vi "ReadTorque-sub.vi"(0 "Torque Setpoint":dbl=1.0 format="%#_13g", 1 "Test Time":dbl, 9 "index 2":i32, 12 "State 2":bool, 13 "State 3":bool) -> (3 "Encoder":dbl[](array[numeric]), 4 "Torque":dbl[](array[numeric]), 5 "Torque":cluster{dbl, dbl}[](array[cluster]), 6 "RPMValue":i32, 8 "Torque vs. Angle":cluster{dbl, dbl}[](array[cluster]), 10 "rpm":cluster{dbl, dbl}[](array[cluster]), 11 "Voltage":cluster{dbl, "voltage out":dbl}[](array[cluster]), 15 "error out":errorcluster)   [LabVIEW 2015]
uses:
  <vilib>/Platform/TimedLoop/XDataNode/timing_clust.ctl
  <vilib>/Platform/TimedLoop/XDataNode/nitl_modes.ctl
  <vilib>/Platform/TimedLoop/XDataNode/wakeup.ctl
  C:/Program Files (x86)/National Instruments/LabVIEW 2015/FUTEK USB DLL.dll
  FUTEK USB DLL.dll
  <vilib>/platform/TimedLoop/XDataNode/XDataNode.xnode
  <vilib>/Platform/TimedLoop/XDataNode/XDNodeRunTimeDep.lvlib
panel:
  out "Array":cluster{dbl, "Torque Error":dbl}[](array[cluster])
  in  "FirstFound":bool=TRUE
  in  "Address":string="1"
  out "Get ADC Sampling RAte 2":string
  out "Get_Decimal Point":string
  out "Get_Fullscale_Load":string
  out "Get_Fullscale_Value":string
  out "Get_Offset_Load":string
  out "Get_Offset_Value":string
  out "get Rotation values 2":string
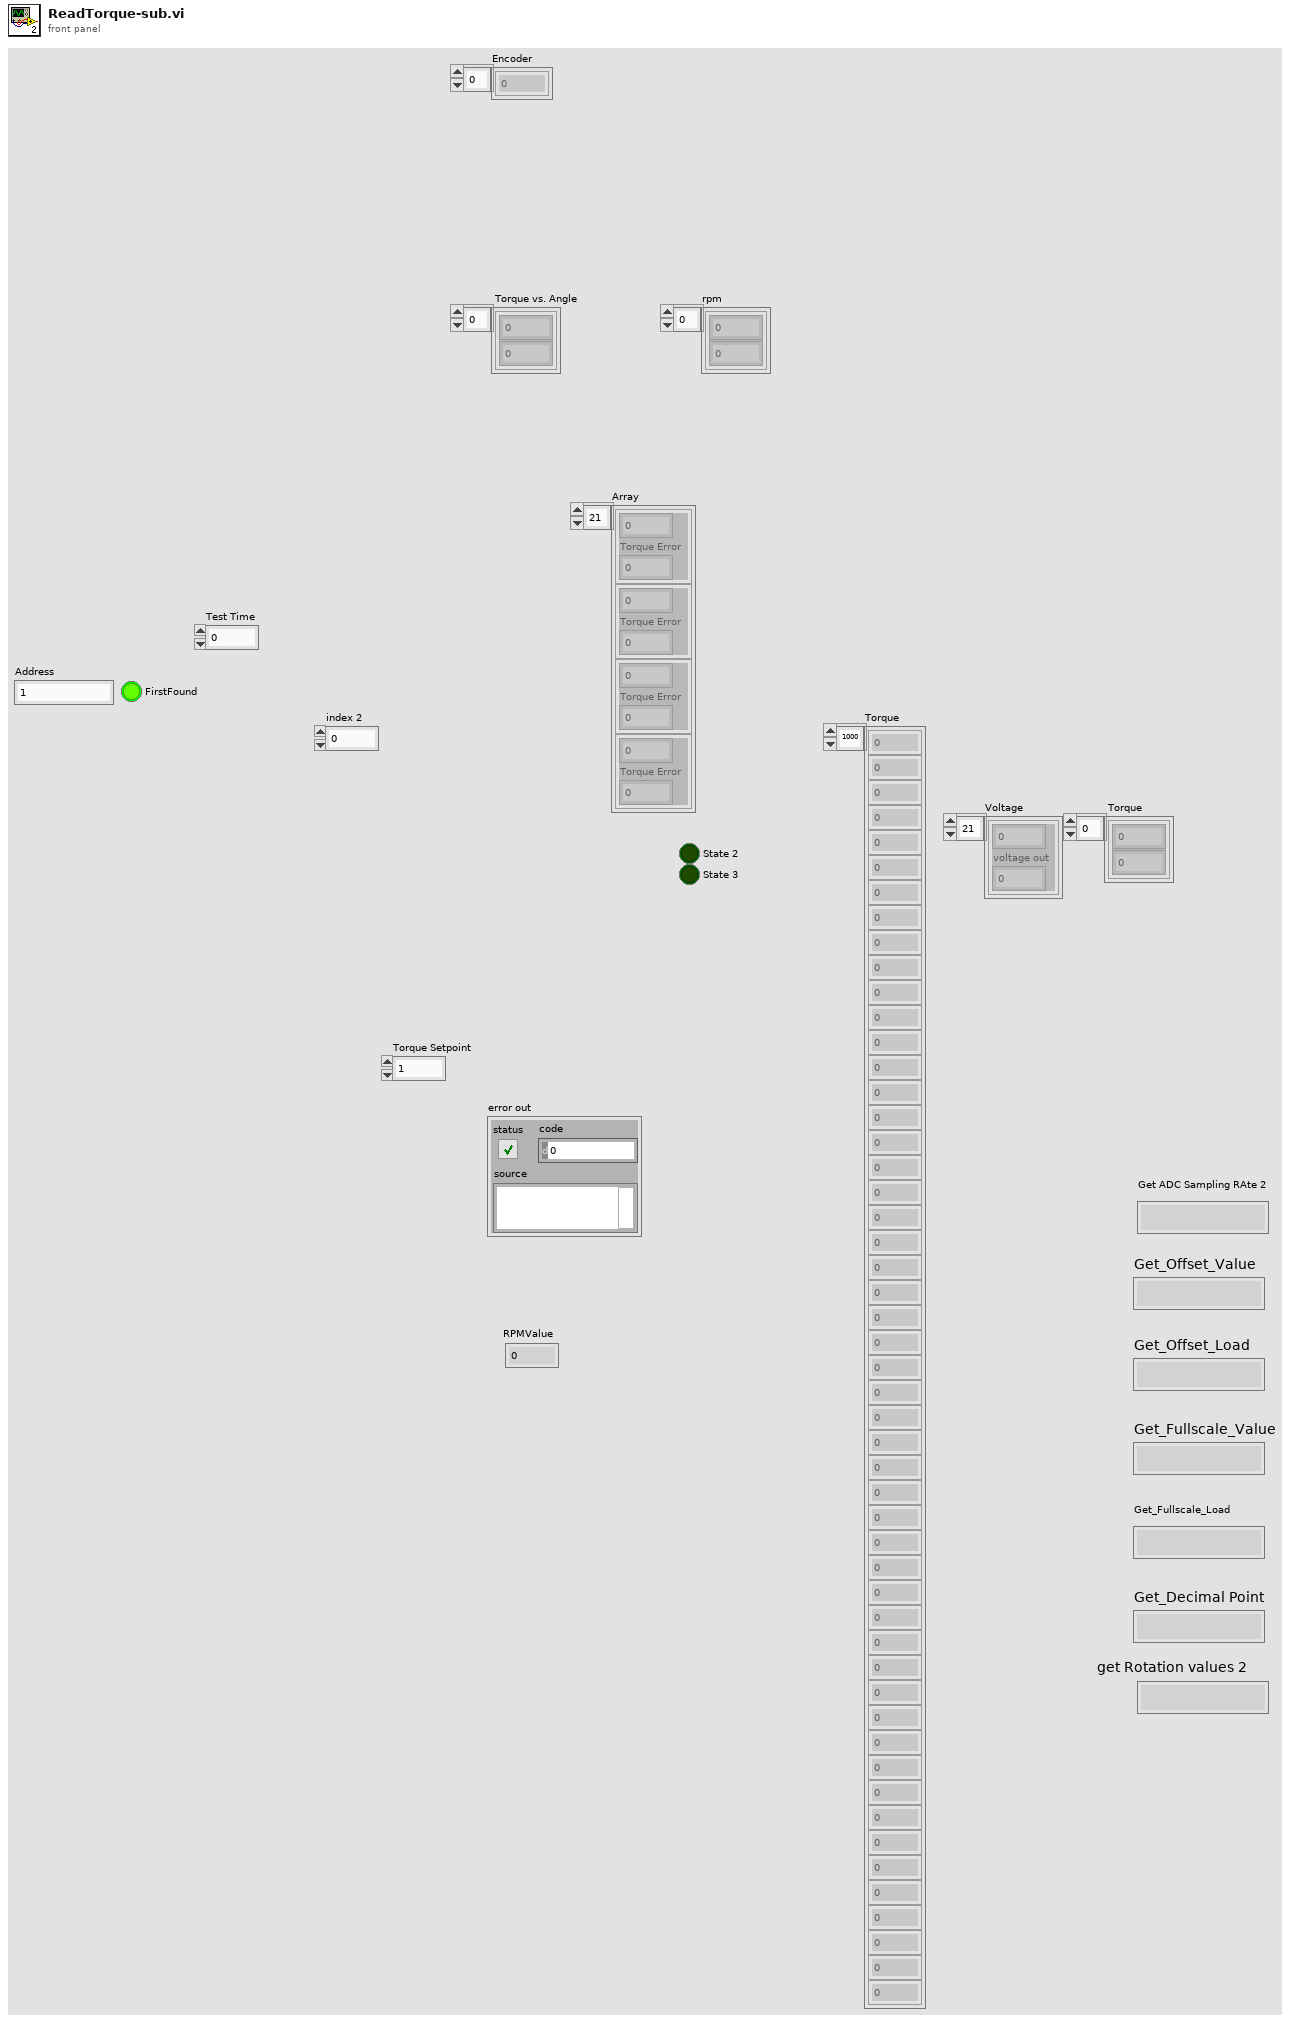
[diagram p1: front panel]
types:
  T1 = typedef "XDNodeRunTimeDep.lvlib/timing_clust.ctl" = cluster{"Expected End [f-1]":u64, "Actual End [f-1]":u64, "Finished Late? [f-1]":bool, "Expected End [i-1]":u64, "Actual End [i-1]":u64, "Finished Late? [i-1]":bool, "Expected Start [i]":u64, "Actual Start [i]":u64, "Expected Start [f]":u64, "Actual Start [f]":u64, "Source Name":string, "Structure Name":string, "Period":i64, "Deadline":i64, "Offset":i64, "Start":i64, "Priority":i32, "Timeout":i32, "Mode":T2, "Wakeup Reason":T3, "Error":errorcluster, "Source Type":string, "Secondary Source Type":string, "Global End Time":u64, "Global Start Time":u64, "Frame Duration":u64, "Iteration Duration":u64, "Assigned CPU":i32, "I/O Scan Engine Mode":u32}
  T2 = typedef "XDNodeRunTimeDep.lvlib/nitl_modes.ctl" = enum32{"No Change", "Process missed periods, maintain original phase", "Discard missed periods, maintain original phase", "Process missed periods, ignore original phase", "Discard missed periods, ignore original phase"}
  T3 = typedef "XDNodeRunTimeDep.lvlib/wakeup.ctl" = enum32{"Normal", "Aborted", "Asynchronous wakeup", "Timing source error", "Timed loop error", "Timeout"}
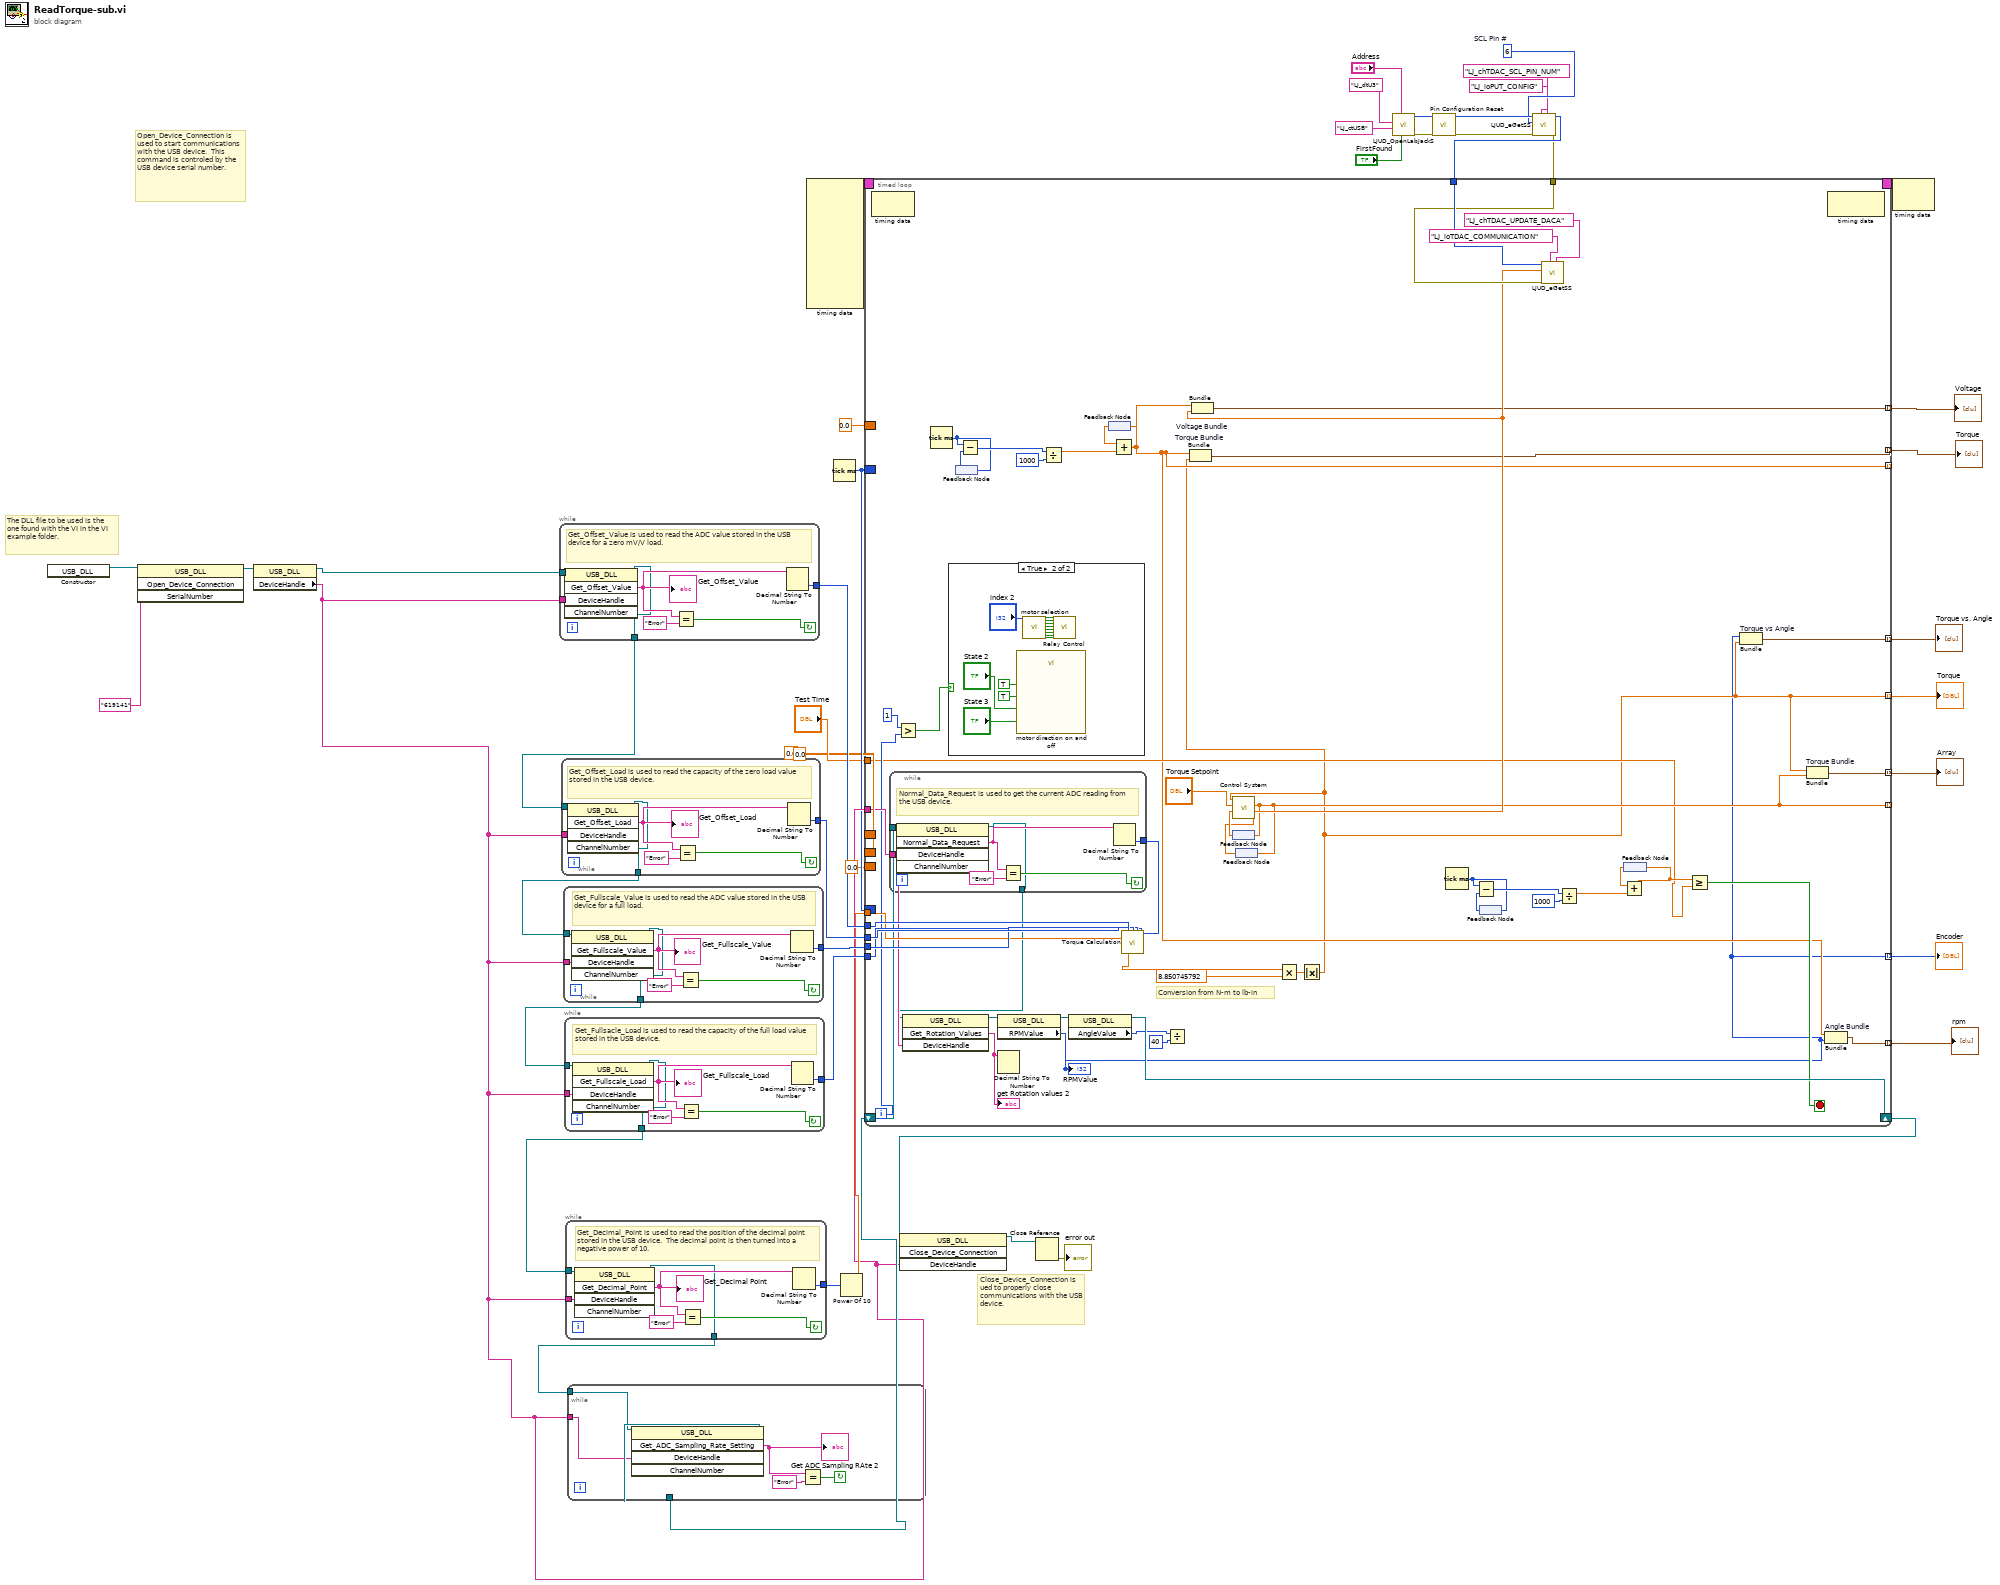
[diagram p0: block diagram]
diagram:
  w26 = 6  # SCL Pin #
  # "The DLL file to be used is the one found with the VI in the VI example folder."
  # "Close_Device_Connection is ued to properly close communications with the USB device."
  # "Open_Device_Connection is used to start communications with the USB device.  This command is controled by the USB device serial number."
  n1 = constructor class="USB_DLL"() -> (reference out=w37:refnum<k24>)  [unwired: 3 in, 2 out]
  n2 = invoke class="USB_DLL" method="Open_Device_Connection"(reference=w37, "SerialNumber"="619141") -> (reference out=w38:refnum<k24>)  [unwired: 2 in, 3 out]
  n3 = property class="USB_DLL"(reference=w38) -> (reference out=w29:refnum<k24>, "DeviceHandle"=w30:string)  [unwired: 1 in, 1 out]
  n4 = while {
    tunnel: w29 -> [w55]
    tunnel: w30 -> [w54]
    tunnel: [w50] -> w46
    tunnel: [w49] -> w41
    stop <- w51 continue-if-true
    # "Get_Offset_Value is used to read the ADC value stored in the USB device for a zero mV/V load."
    n5 = invoke class="USB_DLL" method="Get_Offset_Value"(reference=w55, "DeviceHandle"=w54) -> (reference out=w49:refnum<k24>, "Get_Offset_Value"=w53:string)  [unwired: 3 in, 3 out]
    "Get_Offset_Value" <- w53
    n6 = Equal?(x=w53, y="Error") -> (x = y?=w51:bool)
    n7 = Decimal String To Number(string=w53) -> (number=w50:i32)  [unwired: 2 in, 1 out]
  }
  n8 = while {
    tunnel: [w59] -> w45
    tunnel: [w58] -> w40
    tunnel: w41 -> [w57]
    tunnel: w30 -> [w56]
    stop <- w60 continue-if-true
    # "Get_Offset_Load is used to read the capacity of the zero load value stored in the USB device."
    n9 = invoke class="USB_DLL" method="Get_Offset_Load"(reference=w57, "DeviceHandle"=w56) -> (reference out=w58:refnum<k24>, "Get_Offset_Load"=w62:string)  [unwired: 3 in, 3 out]
    "Get_Offset_Load" <- w62
    n10 = Equal?(x=w62, y="Error") -> (x = y?=w60:bool)
    n11 = Decimal String To Number(string=w62) -> (number=w59:i32)  [unwired: 2 in, 1 out]
  }
  n12 = while {
    tunnel: [w66] -> w44
    tunnel: [w65] -> w39
    tunnel: w40 -> [w64]
    tunnel: w30 -> [w63]
    stop <- w67 continue-if-true
    # "Get_Fullscale_Value is used to read the ADC value stored in the USB device for a full load."
    n13 = invoke class="USB_DLL" method="Get_Fullscale_Value"(reference=w64, "DeviceHandle"=w63) -> (reference out=w65:refnum<k24>, "Get_Fullscale_Value"=w69:string)  [unwired: 3 in, 3 out]
    "Get_Fullscale_Value" <- w69
    n14 = Equal?(x=w69, y="Error") -> (x = y?=w67:bool)
    n15 = Decimal String To Number(string=w69) -> (number=w66:i32)  [unwired: 2 in, 1 out]
  }
  n16 = while {
    tunnel: [w73] -> w43
    tunnel: [w72] -> w33
    tunnel: w39 -> [w71]
    tunnel: w30 -> [w70]
    stop <- w74 continue-if-true
    # "Get_Fullsacle_Load is used to read the capacity of the full load value stored in the USB device."
    n17 = invoke class="USB_DLL" method="Get_Fullscale_Load"(reference=w71, "DeviceHandle"=w70) -> (reference out=w72:refnum<k24>, "Get_Fullscale_Load"=w76:string)  [unwired: 3 in, 3 out]
    "Get_Fullscale_Load" <- w76
    n18 = Equal?(x=w76, y="Error") -> (x = y?=w74:bool)
    n19 = Decimal String To Number(string=w76) -> (number=w73:i32)  [unwired: 2 in, 1 out]
  }
  n20 = while {
    tunnel: [w80] -> w47
    tunnel: w33 -> [w79]
    tunnel: w30 -> [w78]
    tunnel: [w77] -> w32
    stop <- w81 continue-if-true
    # "Get_Decimal_Point is used to read the position of the decimal point stored in the USB device.  The decimal point is then turned into a negative power of 10."
    n21 = invoke class="USB_DLL" method="Get_Decimal_Point"(reference=w79, "DeviceHandle"=w78) -> (reference out=w77:refnum<k24>, "Get_Decimal_Point"=w83:string)  [unwired: 3 in, 3 out]
    "Get_Decimal Point" <- w83
    n22 = Equal?(x=w83, y="Error") -> (x = y?=w81:bool)
    n23 = Decimal String To Number(string=w83) -> (number=w80:i32)  [unwired: 2 in, 1 out]
  }
  n24 = while {
    tunnel: [w86] -> w31
    tunnel: w32 -> [w85]
    tunnel: w30 -> [w84]
    stop <- w87 continue-if-true
    n25 = invoke class="USB_DLL" method="Get_ADC_Sampling_Rate_Setting"(reference=w85, "DeviceHandle"=w84) -> (reference out=w86:refnum<k24>, "Get_ADC_Sampling_Rate_Setting"=w89:string)  [unwired: 3 in, 3 out]
    "Get ADC Sampling RAte 2" <- w89
    n26 = Equal?(x=w89, y="Error") -> (x = y?=w87:bool)
  }
  n27 = node-c288() -> (w10:T1)  [unwired: 10 in]
  n28 = Tick Count (ms)() -> (millisecond timer value=w13:u32)
  n29 = Power Of 10(x=w47) -> (10^x=w42:dbl)
  n30 = call "LJUD_OpenLabJackS.vi"("FirstFound"="FirstFound", "Address"="Address", "ConnectionType"="LJ_ctUSB", "DeviceType"="LJ_dtU3") -> ("error out"=w23:errorcluster, "Handle"=w22:i32)  [unwired: 5 in, 1 out]
  n31 = call "Pin Configuration Reset.vi"("error in"=w23, "Handle In"=w22) -> ("error out"=w28:errorcluster, "Handle Out"=w27:i32)  [unwired: 8 in]
  n32 = call "LJUD_eGetSS.vi"("Channel"="LJ_chTDAC_SCL_PIN_NUM", "IOType"="LJ_ioPUT_CONFIG", "error in"=w28, "Value Write"=w26, "Handle In"=w27) -> ("error out"=w16:errorcluster, "Handle Out"=w17:i32)  [unwired: 4 in, 1 out]
  n33 = timed-loop {
    tunnel: w46 -> [w142]
    tunnel: w45 -> [w141]
    tunnel: w44 -> [w140]
    tunnel: w43 -> [w139]
    tunnel: w42 -> [w138]
    tunnel: w30 -> [w137]
    shift-right: [w136] -> w35
    shift-left: w31 -> [w135]
    tunnel: w17 -> [w117]
    tunnel: w16 -> [w116]
    border: w13 -> [_]
    border: 0.0 -> [_]
    tunnel: [w100] -> w11 mode=indexing
    tunnel: [w109] -> w14 mode=indexing
    border: w13 -> [_]
    border: 0.0 -> [_]
    tunnel: [w92] -> w8 mode=indexing
    tunnel: [w93] -> _ mode=indexing
    timing: w10 -> [_]
    timing-out: [_] -> w9
    tunnel: "Test Time" -> [w95]
    tunnel: [w96] -> _ mode=indexing
    tunnel: [w98] -> w6 mode=indexing
    border: 0.0 ("Torque Error") -> [_]
    border: 0.0 ("Torque Error") -> [_]
    tunnel: [w94] -> w3 mode=indexing
    tunnel: [w90] -> w2 mode=indexing
    tunnel: [w91] -> w1 mode=indexing
    i -> [w121]
    stop <- w101 stop-if-true
    # "Conversion from N-m to lb-in"
    n34 = node-c288() -> ()  [unwired: 1 in, 1 out]
    n35 = while {
      tunnel: [w162] -> w134
      tunnel: w137 -> [w161]
      tunnel: [w159] -> w128
      tunnel: w135 -> [w158]
      stop <- w163 continue-if-true
      # "Normal_Data_Request is used to get the current ADC reading from the USB device."
      n36 = invoke class="USB_DLL" method="Normal_Data_Request"(reference=w158, "DeviceHandle"=w161) -> (reference out=w159:refnum<k24>, "Normal_Data_Request"=w160:string)  [unwired: 3 in, 3 out]
      n37 = Equal?(x=w160, y="Error") -> (x = y?=w163:bool)
      n38 = Decimal String To Number(string=w160) -> (number=w162:i32)  [unwired: 2 in, 1 out]
    }
    n39 = Greater?(x=1, y=w121) -> (0:w122:bool)
    n40 = invoke class="USB_DLL" method="Get_Rotation_Values"(reference=w128, "DeviceHandle"=w137) -> (reference out=w130:refnum<k24>, "Get_Rotation_Values"=w131:string)  [unwired: 2 in, 2 out]
    "get Rotation values 2" <- w131
    n41 = Tick Count (ms)() -> (millisecond timer value=w112:u32)
    n42 = case shown="True" w122 {
      frame False {
      }
      frame True {
        n43 = call "motor direction on and off.vi"("State 3"="State 3", "State 2"="State 2", "State 1"=TRUE, "State 0"=TRUE) -> ()  [unwired: 8 in]
        n44 = call "motor selection.vi"("index 2"="index 2") -> ("[0]"=w146:bool, "[1]"=w147:bool, "[2]"=w148:bool, "[3]"=w149:bool, "[4]"=w150:bool, "[5]"=w151:bool, "[6]"=w152:bool, "[7]"=w153:bool)  [unwired: 19 in]
        n45 = call "Relay Control.vi"("State 8"=w146, "State 9"=w147, "State 10"=w148, "State 11"=w149, "State 12"=w150, "State 13"=w151, "State 14"=w152, "State 15"=w153) -> ()  [unwired: 20 in]
      }
    }
    n46 = feedback #1() -> (w113:u32)
    n47 = feedback-in #1(w112) -> ()
    n48 = Subtract(x=w112, y=w113) -> (x-y=w114:u32)
    n49 = property class="USB_DLL"(reference=w130) -> (reference out=w129:refnum<k24>, "RPMValue"=w90:i32)  [unwired: 1 in, 1 out]
    "RPMValue" <- w90
    n50 = Decimal String To Number(string=w131) -> ()  [unwired: 2 in, 2 out]
    n51 = Divide(x=w114, y=u32 1000) -> (x/y=w99:dbl)
    n52 = property class="USB_DLL"(reference=w129) -> (reference out=w136:refnum<k24>, "AngleValue"=w127:i32)  [unwired: 1 in, 1 out]
    n53 = feedback #2() -> (w111:dbl)
    n54 = Add(x=w111, y=w99) -> (x+y=w93:dbl)
    n55 = feedback-in #2(w93) -> ()
    n56 = call "Torque Calculation.vi"("Normal_Data_Request"=w134, "Get_Offset_Value"=w142, "Get_Offset_Load"=w141, "Get_Fullscale_Value"=w140, "Get_Fullscale_Load"=w139, "Get_Decimal_Point"=w138) -> ("Result"=w132:dbl)  [unwired: 8 in, 1 out]
    n57 = Divide(x=w127, y=40) -> ()  [unwired: 1 out]
    n58 = feedback #3() -> (w125:dbl)
    n59 = feedback #4() -> (w97:dbl)
    n60 = Multiply(x=w132, y=8.850745792) -> (x*y=w123:dbl)
    n61 = Absolute Value(x=w123) -> (abs(x)=w92:dbl)
    n62 = Bundle "Torque Bundle"(w93, w92) -> (w100:cluster{dbl, dbl})  [unwired: 1 in]
    n63 = call "Control System.vi"("last torque value"=w97, "Sum of error"=w125, "Torque Setpoint"="Torque Setpoint", "Torque  Read"=w92) -> ("voltage out"=w110:dbl, "Torque Error"=w96:dbl)  [unwired: 6 in]
    n64 = Bundle "Voltage Bundle"(w93, "voltage out"=w110) -> (w109:cluster{dbl, "voltage out":dbl})  [unwired: 1 in]
    n65 = feedback-in #3(w96) -> ()
    n66 = feedback-in #4(w96) -> ()
    n67 = Tick Count (ms)() -> (millisecond timer value=w105:u32)
    n68 = feedback #5() -> (w106:u32)
    n69 = Subtract(x=w105, y=w106) -> (x-y=w107:u32)
    n70 = feedback-in #5(w105) -> ()
    n71 = call "LJUD_eGetSS.vi"("Channel"="LJ_chTDAC_UPDATE_DACA", "IOType"="LJ_ioTDAC_COMMUNICATION", "error in"=w116, "Value Write"=w110, "Handle In"=w117) -> ()  [unwired: 4 in, 3 out]
    n72 = Divide(x=w107, y=u32 1000) -> (x/y=w104:dbl)
    n73 = feedback #6() -> (w103:dbl)
    n74 = Add(x=w103, y=w104) -> (x+y=w102:dbl)
    n75 = feedback-in #6(w102) -> ()
    n76 = Greater Or Equal?(x=w102, y=w95) -> (x >= y?=w101:bool)
    n77 = Bundle "Torque vs Angle"("RPMValue"=w90, w92) -> (w91:cluster{"RPMValue":i32, dbl})  [unwired: 1 in]
    n78 = Bundle "Torque Bundle"(w92, "Torque Error"=w96) -> (w98:cluster{dbl, "Torque Error":dbl})  [unwired: 1 in]
    n79 = Bundle "Angle Bundle"(w93, "RPMValue"=w90) -> (w94:cluster{dbl, "RPMValue":i32})  [unwired: 1 in]
    n80 = node-c288() -> ()  [unwired: 1 in, 1 out]
  }
  "Voltage" <- w14
  "Torque" <- w11
  "Torque" <- w8
  "Array" <- w6
  "rpm" <- w3
  "Encoder" <- w2
  "Torque vs. Angle" <- w1
  n81 = invoke class="USB_DLL" method="Close_Device_Connection"(reference=w35, "DeviceHandle"=w30) -> (reference out=w48:refnum<k24>)  [unwired: 2 in, 3 out]
  n82 = Close Reference(reference=w48) -> (error out=→"error out":errorcluster)  [unwired: 1 in]
  n83 = node-c288(w9) -> ()  [unwired: 1 out]
